vi "Swerve Motor Back Left.vi"(0 "Steer motor reference name":string="My Motor RefNum", 1 "Drive motor reference name":string="My Motor RefNum", 2 "Speed command":dbl, 3 "Direction command (deg)":dbl) -> ()   [LabVIEW 2018]
uses:
  <vilib>/Rock Robotics/WPI/ThirdParty/REV Robotics/SPARK MAX/Typedef/Spark MAX Control Type.ctl
  <vilib>/Rock Robotics/WPI/ThirdParty/Phoenix-LabVIEW/Motor Controller/Controls/CTRE_Phoenix_MotorControl_ControlMode.ctl
  <vilib>/Rock Robotics/WPI/ThirdParty/Phoenix-LabVIEW/Motor Controller/Get/CTRE_Phoenix_MotorController_GetAnalogData.vi
  <vilib>/Rock Robotics/WPI/ThirdParty/Phoenix-LabVIEW/Motor Controller/Get/CTRE_Phoenix_MotorController_GetSelectedSensorData.vi
  Robot Global Data.vi
panel:
  in  "Numeric":dbl
  out "Position (Raw Sensor Units) 2":i32
  out "AnalogInWithOv":i32
  out "New Position":dbl
  out "Flip motors?":bool
  out "Degres To Travel":dbl
  out "Better Angle 2":dbl(knob)=41.7137932364482 scale=0.0..360.0
  in  "Ramp Rate-BL":dbl=60.0
  in  "I Zone-BL":dbl
  in  "F-BL":dbl=0.25
  in  "D-BL":dbl=0.5
  in  "I-BL":dbl=0.001
  in  "P-BL":dbl=4.0
  out "Veloicity":dbl
  out "Back Left Angle":dbl
  out "Position (Raw Sensor Units)":i32
  # "VI inputs"
  # "Intermediate values"
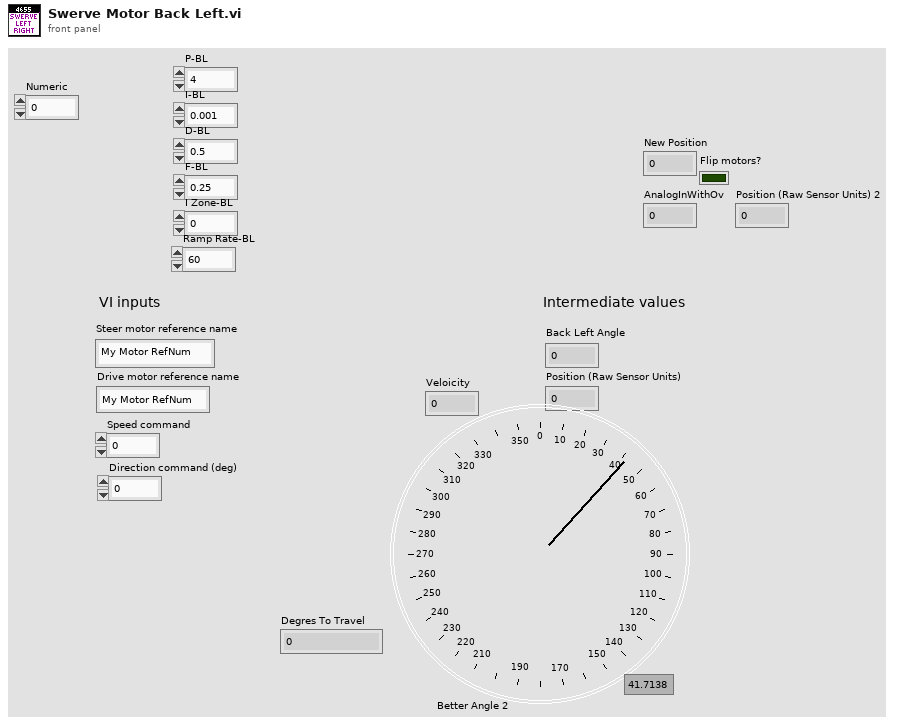
[diagram p1: front panel]
types:
  T1 = typedef "Spark MAX Control Type.ctl" = enum16{"Percent VBus", "Voltage", "Velocity", "Position", "Smart Motion", "Current", "Smart Velocity"}
  T2 = typedef "WPI_MotorControlDeviceRef.ctl" = cluster{"DeviceStatus":errorcluster, "Type":T3, "PWM":cluster{"PWM Channel":T4, "DeadBand":T5}, "CAN":cluster{"Device Number":u8, "SetOutput VI Ref":variant, "GetOutput VI Ref":variant, "Enable VI Ref":variant, "Disable VI Ref":variant, "Data":variant}, "Invert":bool, "DIO PWM":cluster{"PWM \"Enable\" Channel":T4, "DIOChannel":T6, "PWM Rate":dbl}}
  T3 = typedef "WPI_MotorControlType.ctl" = enum16{"PWM", "CAN", "DIO PWM"}
  T4 = typedef "FPGA_DIOPWMChannel.ctl" = enum8{"PWM 0", "PWM 1", "PWM 2", "PWM 3", "PWM 4", "PWM 5", "PWM 6", "PWM 7", "PWM 8", "PWM 9", "PWM MXP 0", "PWM MXP 1", "PWM MXP 2", "PWM MXP 3", "PWM MXP 4", "PWM MXP 5", "PWM MXP 6", "PWM MXP 7", "PWM MXP 8", "PWM MXP 9", "Invalid"}
  T5 = typedef "WPI_PWMDeadband.ctl" = cluster{"Name":string, "maxPositivePwm":i32, "minPositivePwm":i32, "centerPwm":i32, "maxNegativePwm":i32, "minNegativePwm":i32, "angularRange":u16}
  T6 = typedef "FPGA_DIOChannel.ctl" = enum8{"DIO 0", "DIO 1", "DIO 2", "DIO 3", "DIO 4", "DIO 5", "DIO 6", "DIO 7", "DIO 8", "DIO 9", "DIO MXP 0", "DIO MXP 1", "DIO MXP 2", "DIO MXP 3", "DIO MXP 4", "DIO MXP 5", "DIO MXP 6", "DIO MXP 7", "DIO MXP 8", "DIO MXP 9", "DIO MXP 10", "DIO MXP 11", "DIO MXP 12", "DIO MXP 13", "DIO MXP 14", "DIO MXP 15", "SPI Port CS1", "SPI Port CS2", "SPI Port CS3", "SPI Port MISO", "SPI Port MOSI", "Invalid"}
  T7 = typedef "CTRE_Phoenix_MotorControl_ControlMode.ctl" = u16
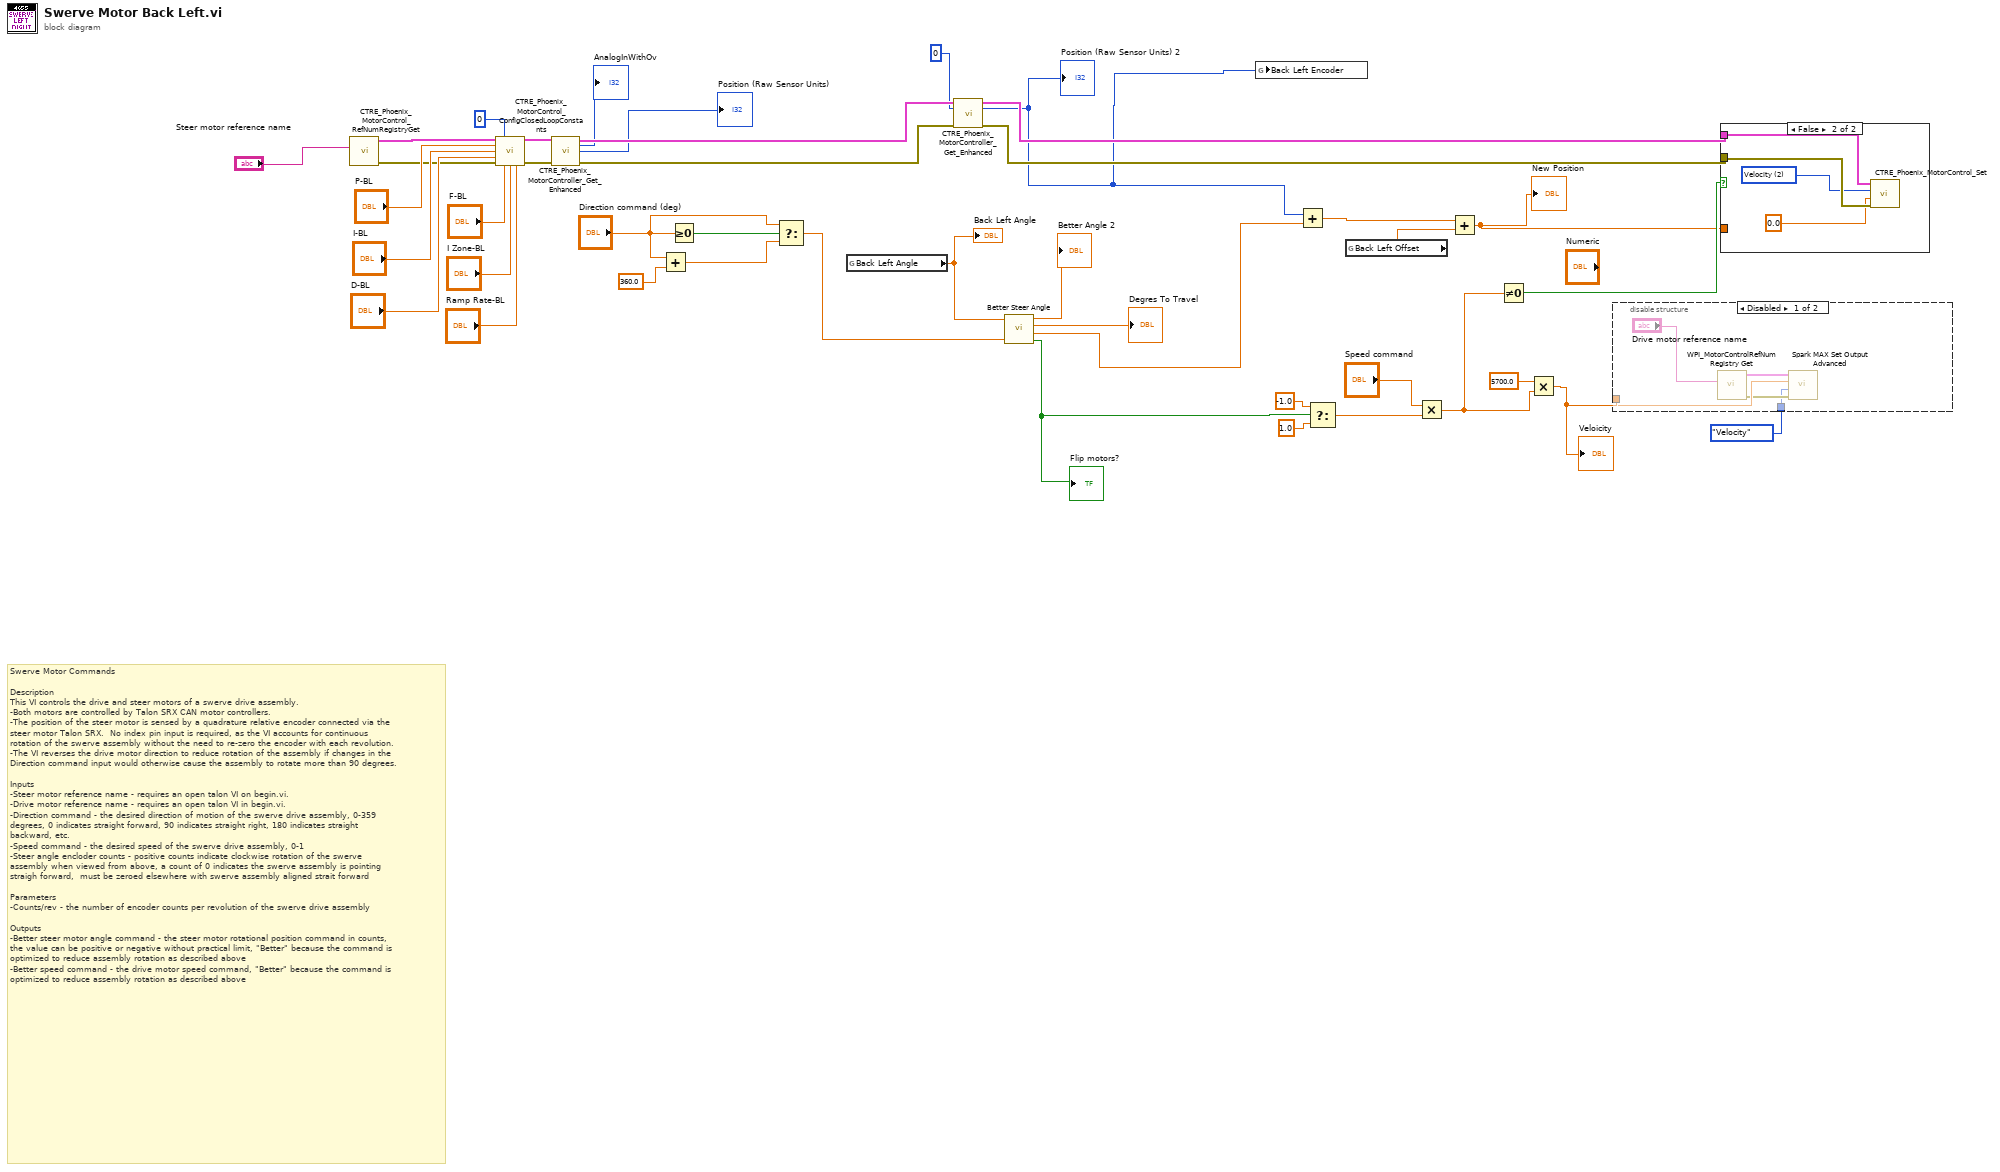
[diagram p0: block diagram]
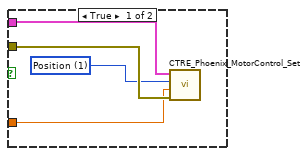
[diagram p3: hidden frame]
diagram:
  # "Swerve Motor Commands\n\nDescription\nThis VI controls the drive and steer motors of a swerve drive assembly.  \n-Both motors are controlled by Talon SRX CAN motor controllers.  \n-The position of the steer motor is sensed by a quadrature relative encoder connected via the steer motor Talon SRX.  No index pin input is required, as the VI accounts for continuous rotation of the swerve assembly without the need to re-zero the encoder with each revolution.\n-The VI reverses the drive motor direction to reduce rotation of the assembly if changes in the Direction command input would otherwise cause the assembly to rotate more than 90 degrees.\n\nInputs\n-Steer motor reference name - requires an open talon VI on begin.vi.\n-Drive motor reference name - requires an open talon VI in begin.vi.\n-Direction command - the desired direction of motion of the swerve drive assembly, 0-359 degrees, 0 indicates straight forward, 90 indicates straight right, 180 indicates straight backward, etc.\n-Speed command - the desired speed of the swerve drive assembly, 0-1\n-Steer angle encloder counts - positive counts indicate clockwise rotation of the swerve assembly when viewed from above, a count of 0 indicates the swerve assembly is pointing straigh forward,  must be zeroed elsewhere with swerve assembly aligned strait forward\n\nParameters\n-Counts/rev - the number of encoder counts per revolution of the swerve drive assembly\n\nOutputs\n-Better steer motor angle command - the steer motor rotational position command in counts, the value can be positive or negative without practical limit, \"Better\" because the command is optimized to reduce assembly rotation as described above\n-Better speed command - the drive motor speed command, \"Better\" because the command is optimized to reduce assembly rotation as described above"
  n1 = call <vilib>:"CTRE_Phoenix_MotorControl_RefNumRegistryGet.vi"("refnum name"="Steer motor reference name") -> ("error out"=w23:errorcluster, "PhoenixMotorControlDevRef"=w24:T2)  [unwired: 9 in]
  n2 = call <vilib>:"CTRE_Phoenix_MotorControl_ConfigClosedLoopConstants.vi"("PhoenixMotorControlDevRef"=w24, "slotIdx"=0, "P"="P-BL", "I"="I-BL", "D"="D-BL", "error in (no error)"=w23, "F"="F-BL", "I Zone"="I Zone-BL", "timeoutMs"="Ramp Rate-BL") -> ("PhoenixMotorControlDevRef"=w28:T2, "error out"=w27:errorcluster)  [unwired: 5 in]
  n3 = call-poly <vilib>:"CTRE_Phoenix_MotorController_Get_Enhanced.vi"("PhoenixMotorControlDevRef"=w28, "error in"=w27) -> ("PhoenixMotorControlDevRef"=w11:T2, "AnalogInWithOv"=→"AnalogInWithOv":i32, "AnalogInRaw"=→"Position (Raw Sensor Units)":i32, "error out"=w9:errorcluster)  [unwired: 9 in, 1 out]
  n4 = Add(x="Direction command (deg)", y=360.0) -> (x+y=w20:dbl)
  n5 = Greater Or Equal To 0?(x="Direction command (deg)") -> (x >= 0?=w22:bool)
  n6 = Select(t="Direction command (deg)", s=w22, f=w20) -> (s? t:f=w16:dbl)
  n7 = global read "Robot Global Data.vi" "Back Left Angle"() -> (w17:dbl)
  "Back Left Angle" <- w17
  n8 = call-poly <vilib>:"CTRE_Phoenix_MotorController_Get_Enhanced.vi"("PhoenixMotorControlDevRef"=w11, "pidLoopIdx"=u32 0, "error in"=w9) -> ("PhoenixMotorControlDevRef"=w10:T2, "Position (Raw Sensor Units)"=w1:i32, "error out"=w8:errorcluster)  [unwired: 9 in, 1 out]
  "Position (Raw Sensor Units) 2" <- w1
  n9 = call "Better Steer Angle.vi"("Current Angle"=w17, "Set Point"=w16) -> ("Better Angle"=→"Better Angle 2":dbl, "Degres To Travel"=→"Degres To Travel":dbl, "Encoder Count to Move"=w3:dbl, "Flip motors?"=w14:bool)  [unwired: 1 in]
  "Flip motors?" <- w14
  n10 = global write "Robot Global Data.vi" "Back Left Encoder"(w1) -> ()
  n11 = Add(x=w1, y=w3) -> (x+y=w13:dbl)
  n12 = Select(t=-1.0, s=w14, f=1.0) -> (s? t:f=w40:dbl)
  n13 = global read "Robot Global Data.vi" "Back Left Offset"() -> (w18:dbl)
  n14 = Multiply(x="Speed command", y=w40) -> (x*y=w35:dbl)
  n15 = Add(x=w13, y=w18) -> (x+y=w5:dbl)
  "New Position" <- w5
  n16 = Not Equal To 0?(x=w35) -> (x != 0?=w36:bool)
  n17 = Multiply(x=5700.0, y=w35) -> (x*y=w37:dbl)
  "Veloicity" <- w37
  n18 = disable-structure shown="Disabled" {
    disable-tunnel: w37 -> [w47 _]
    disable-tunnel: Spark_MAX_Control_Type."Velocity" ("Control Mode") -> [w44 _]
    frame Disabled {
      n19 = call <vilib>:"WPI_MotorControlRefNum Registry Get.vi"("refnum name"="Drive motor reference name") -> ("error out"=w46:errorcluster, "MotorControlDevRef"=w45:T2)  [unwired: 9 in]
      n20 = call <vilib>:"Spark MAX Set Output Advanced.vi"("error in (no error)"=w46, "Control Mode"=w44, "Setpoint"=w47, "MotorControlDevRef"=w45) -> ()  [unwired: 6 in, 2 out]
    }
    frame Enabled {
    }
  }
  n21 = case shown="False" w36 {
    tunnel: w10 -> [w51 w55]
    tunnel: w8 -> [w50 w54]
    tunnel: w5 -> [w49 _]
    frame True {
      w48 = T7 1 items=["PercentOutput"=0, "Position"=1, "Velocity"=2, "Current"=3, "Follower"=5, "MotionProfile"=6, "MotionMagic"=7, "MotionProfileArc"=10, "Disabled"=15] ("Control Mode")
      n22 = call <vilib>:"CTRE_Phoenix_MotorControl_Set.vi"("error in (no error)"=w50, "Output"=w49, "Control Mode"=w48, "PhoenixMotorControlDevRef"=w51) -> ()  [unwired: 6 in, 2 out]
    }
    frame False {
      w53 = T7 2 items=["PercentOutput"=0, "Position"=1, "Velocity"=2, "Current"=3, "Follower"=5, "MotionProfile"=6, "MotionMagic"=7, "MotionProfileArc"=10, "Disabled"=15] ("Control Mode")
      n23 = call <vilib>:"CTRE_Phoenix_MotorControl_Set.vi"("error in (no error)"=w54, "Output"=0.0 ("y"), "Control Mode"=w53, "PhoenixMotorControlDevRef"=w55) -> ()  [unwired: 6 in, 2 out]
    }
  }
